vi "GetTvalue.vi"(6 "error in":errorcluster caption="错误输入（无错误）", 8 "Numeric":i32, 9 "Pages":refnum<vi>[](array[refnum])) -> (0 "error out":errorcluster caption="错误输出", 3 "T (K) or R":string)   [LabVIEW 2017]
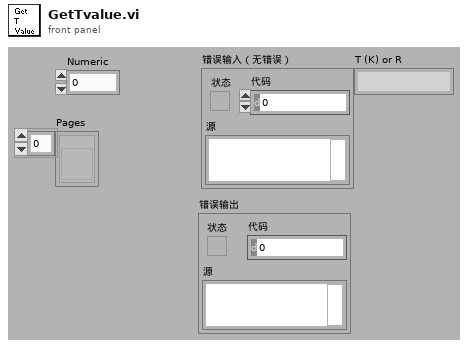
[diagram p1: front panel]
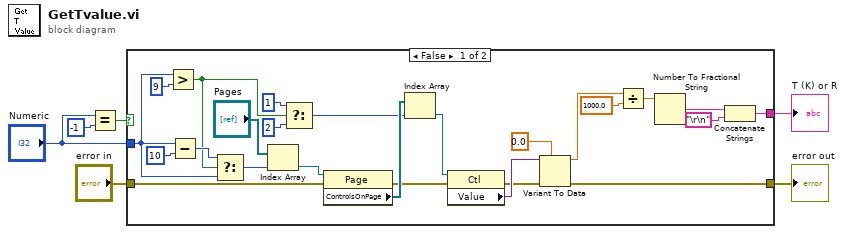
[diagram p0: block diagram]
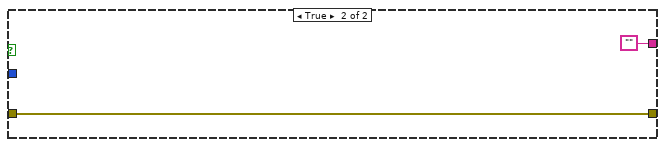
[diagram p2: hidden frame]
diagram:
  n1 = Equal?(x="Numeric", y=-1) -> (x = y?=w5:bool)
  n2 = case shown="False" w5 {
    tunnel: "error in" -> [w23 w33]
    tunnel: "Numeric" -> [w14 _]
    tunnel: [w20 w33] -> w4
    tunnel: [w16 ""] -> w3
    frame False {
      n3 = Greater?(x=w14, y=9) -> (0:w10:bool)
      n4 = Subtract(x=w14, y=10) -> (x-y=w12:i32)
      n5 = Select(t=w12, s=w10, f=w14) -> (s? t:f=w11:i32)
      n6 = Index Array(array="Pages", index=w11) -> (element=w25:refnum<vi>)
      n7 = Select(t=1, s=w10, f=2 ("索引")) -> (s? t:f=w7:i32)
      n8 = property class="Page"(reference=w25, error in=w23) -> (error out=w22:errorcluster, "ControlsOnPage"=w26:refnum<vi>[])  [unwired: 1 out]
      n9 = Index Array(array=w26, index=w7) -> (element=w27:refnum<vi>)
      n10 = property class="Ctl"(reference=w27, error in=w22) -> (error out=w21:errorcluster, "Value"=w28:variant)  [unwired: 1 out]
      n11 = Variant To Data(error in=w21, type=0.0, Variant=w28) -> (data=w30:dbl, error out=w20:errorcluster)
      n12 = Divide(x=w30, y=1000.0) -> (x/y=w17:dbl)
      n13 = Number To Fractional String(number=w17) -> (F-format string=w19:string)  [unwired: 3 out]
      n14 = Concatenate Strings(w19, "\r\n") -> (w16:string)
    }
    frame True {
    }
  }
  "error out" <- w4
  "T (K) or R" <- w3
